vi "DescalePoint.vi"(8 "Y":i32, 9 "X":i32, 10 "Offset":cluster{"x":dbl, "y":dbl}, 11 "Scale":dbl) -> (0 "Y-Out":dbl, 1 "X-Out":dbl)   [LabVIEW 2020, in "LcPictureBox.lvclass"]
uses:
  LcPictureBox.lvclass
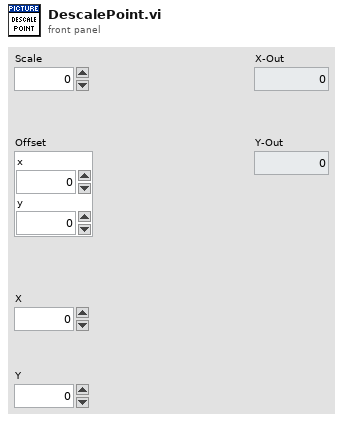
[diagram p1: front panel]
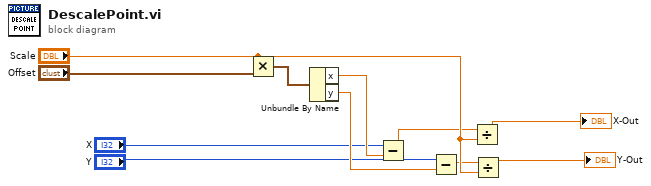
[diagram p0: block diagram]
diagram:
  n1 = Multiply(x="Scale", y="Offset") -> (x*y=w1:cluster{"x":dbl, "y":dbl})
  n2 = Unbundle By Name(w1) -> ("x"=w4:dbl, "y"=w6:dbl)
  n3 = Subtract(x="X", y=w4) -> (x-y=w7:dbl)
  n4 = Subtract(x="Y", y=w6) -> (x-y=w8:dbl)
  n5 = Divide(x=w7, y="Scale") -> (x/y=→"X-Out":dbl)
  n6 = Divide(x=w8, y="Scale") -> (x/y=→"Y-Out":dbl)
